vi "Initialize.vi"(8 "error in (no error)":errorcluster, 11 "UDP in":refnum<class "UDP.lvclass">) -> (0 "error out":errorcluster, 3 "UDP out":refnum<class "UDP.lvclass">)   [LabVIEW 2013, in "Protocol Classes.lvlib" / "UDP.lvclass"]
uses:
  UDP.lvclass
  Protocol Parent/Protocol Parent.lvclass
  UDP.lvclass/UDP.ctl
  Data Access/Read Local IP Address.vi
  Data Access/Read Local Port.vi
  Data Access/Write UDP Ref.vi
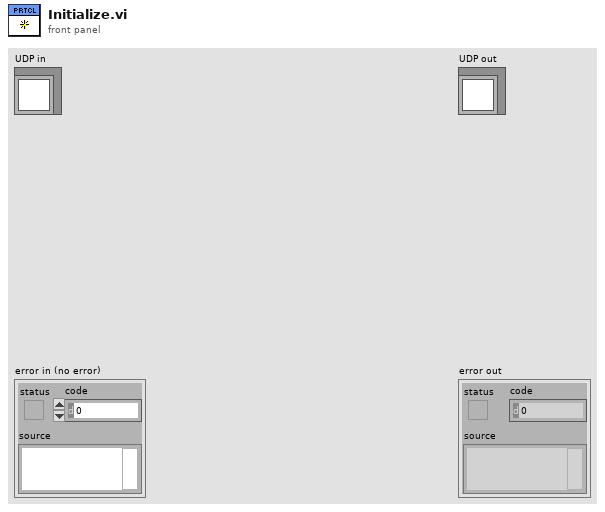
[diagram p1: front panel]
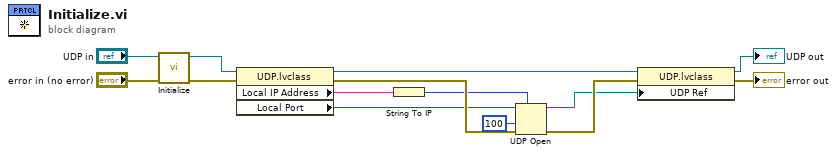
[diagram p0: block diagram]
diagram:
  n1 = call-parent "Initialize.vi"("error in (no error)"="error in (no error)", "Protocol Parent in"="UDP in") -> ("error out"=w12:errorcluster, "Protocol Parent out"=w11:refnum<class "UDP.lvclass">)  [unwired: 8 in]
  n2 = property class="UDP.lvclass"(reference=w11, error in=w12) -> (reference out=w3:refnum<class "UDP.lvclass">, error out=w10:errorcluster, "Local IP Address"=w9:string, "Local Port"=w7:u16)
  n3 = String To IP(1:w9) -> (0:w8:u32)
  n4 = UDP Open(7:w8, 8:w10, 9:100 ("timeout ms (25000)"), 11:w7) -> (port=w1:refnum<k16>, 0:w5:errorcluster)  [unwired: 1 in, 1 out]
  n5 = property class="UDP.lvclass"(reference=w3, error in=w5, "UDP Ref"=w1) -> (reference out=→"UDP out":refnum<class "UDP.lvclass">, error out=→"error out":errorcluster)
